vi "Engine - Diesel - EGR Actuation Host.vi"() -> ()   [LabVIEW 2015, in "ECS-Host.lvlib"]
uses:
  ECS-Host.lvlib
  <vilib>/addons/Software Calibration Management/XControls/TBL1D.xctl
panel:
  out "LowPEGRPsnStp":sgl caption="[%Open]"
  out "LowPEGRDutyCyc_TblOut":sgl caption="[%]"
  out "LowPEGRDutyCyc_Des":sgl caption="[%]"
  in  "LowPEGRDutyCyc_Tbl":cluster{"X":sgl[], "Y":sgl[]}(xcontrol)
  in  "LowPEGRDutyCyc_ManE":bool
  in  "LowPEGRDutyCyc_Man":sgl caption="[%]"
  in  "LowPEGRDutyCyc_Min":sgl caption="[%]"
  in  "LowPEGRDutyCyc_Max":sgl caption="[%]"
  out "HighPEGRPsnStp":sgl caption="[%Open]"
  # "High Pressure EGR Actuator - See Throttle Setup"
  # "Low Pressure EGR (LP-EGR) Actuator"
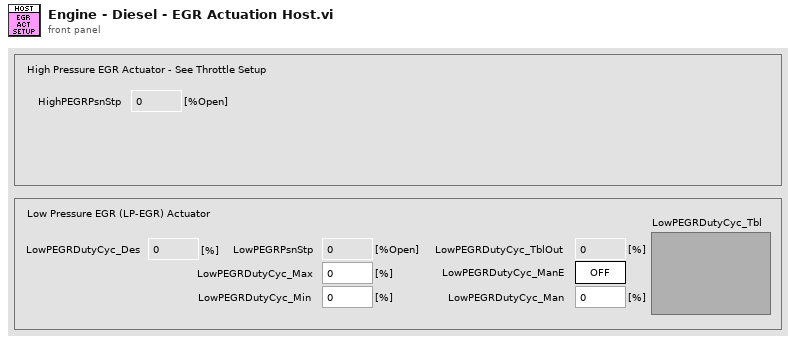
[diagram p1: front panel]
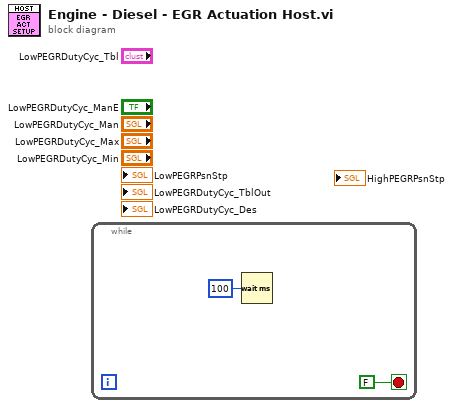
[diagram p0: block diagram]
diagram:
  n1 = while {
    stop <- FALSE stop-if-true
    n2 = Wait (ms)(milliseconds to wait=u32 100) -> ()  [unwired: 1 out]
  }
